vi "MessageDequeue.vi"(8 "error in (no error)":errorcluster, 11 "Input Queue":refnum<queue>) -> (0 "error out":errorcluster, 2 "Message":string, 3 "Input Queue (dup)":refnum<queue>)   [LabVIEW 2018]
panel:
  # "Message Dequeue:\n\nRemoves a message from the queue.\nIf there are no queued messages,\nreturns the last message to arrive"
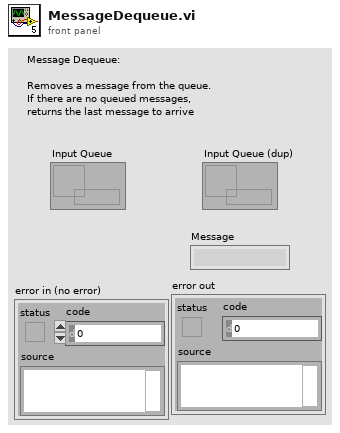
[diagram p1: front panel]
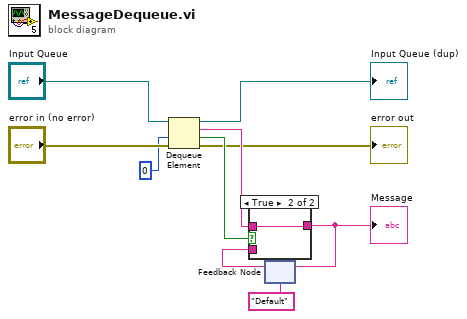
[diagram p0: block diagram]
diagram:
  n1 = Dequeue Element(queue="Input Queue", timeout in ms (-1)=0, error in (no error)="error in (no error)") -> (queue out=→"Input Queue (dup)":refnum<queue>, element=w8:string, timed out?=w9:bool, error out=→"error out":errorcluster)
  n2 = feedback #1("Default") -> (w5:string)
  n3 = case shown="True" w9 {
    tunnel: w8 -> [_ w12]
    tunnel: [w11 w12] -> w6
    tunnel: w5 -> [w11 _]
    frame False {
    }
    frame True {
    }
  }
  "Message" <- w6
  n4 = feedback-in #1(w6) -> ()
